vi "Get BuildSpec Version.vi"(8 "error in (no error)":errorcluster, 11 "Task in":refnum<class "Task.lvclass">) -> (0 "error out":errorcluster, 2 "BuildSpec Version":string, 3 "Task out":refnum<class "Task.lvclass">)   [LabVIEW 2017, in "Task Interface.lvlib" / "Task.lvclass"]
uses:
  Task.lvclass
  Task.lvclass/Task.ctl
  <vilib>/AppBuilder/AB_API_Simple/Get Build Specification Version (path).vi
  <vilib>/AppBuilder/AB_API_Simple/NI_App_Builder_API.lvlib
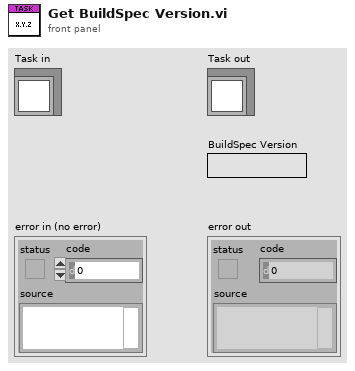
[diagram p1: front panel]
types:
  T1 = typedef "NI_App_Builder_API.lvlib/Build Specification Version.ctl" = cluster{"Major":u16, "Minor":u16, "Fix":u16, "Build":u16}
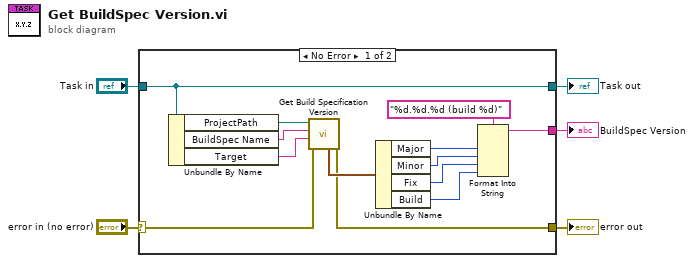
[diagram p0: block diagram]
diagram:
  n1 = case shown="No Error" "error in (no error)" {
    selector: "error in (no error)" -> [w7 w20]
    tunnel: [w6 w20] -> w4
    tunnel: [w18 w19] -> w2
    tunnel: "Task in" -> [w18 w19]
    tunnel: [w12 _] -> w1
    frame No Error {
      n2 = Unbundle By Name(w18) -> ("ProjectPath"=w11:path, "BuildSpec Name"=w10:string, "Target"=w9:string)
      n3 = call-poly <vilib>:"Get Build Specification Version.vi"("error in (no error)"=w7, "Name of target (My Computer)"=w9, "Name of build specification"=w10, "Path to project"=w11) -> ("error out"=w6:errorcluster, "Build Specification Version"=w8:T1)  [unwired: 6 in]
      n4 = Unbundle By Name(w8) -> ("Major"=w17:u16, "Minor"=w16:u16, "Fix"=w15:u16, "Build"=w14:u16)
      n5 = Format Into String(format string="%d.%d.%d (build %d)", w17, w16, w15, w14) -> (resulting string=w12:string)  [unwired: 2 in, 1 out]
    }
    frame Error {
    }
  }
  "error out" <- w4
  "Task out" <- w2
  "BuildSpec Version" <- w1
